vi "Append List to Report.vi"(0 "report in":refnum<class "NI_report.lvclass">, 1 "ordered item type (default)":T1(ring), 2 "unordered item type (default)":enum16{"(default)", "disc", "square", "circle"}(ring), 7 "list elements":string[](array[string]), 9 "list type (ordered)":enum16{"unordered", "ordered"}(ring)=enum."ordered", 11 "error in (no error)":errorcluster, 12 "ordered start (1)":i32=1, 13 "bookmark (Word)":string) -> (4 "report out":refnum<class "NI_report.lvclass">, 8 "start out (Word)":i32, 10 "end out (Word)":i32, 15 "error out":errorcluster)   [LabVIEW 2015, in "NI_report.lvclass"]
doc: "Adds a list of elements to the report."
uses:
  <vilib>/Utility/NIReport.llb/NI_report.lvclass
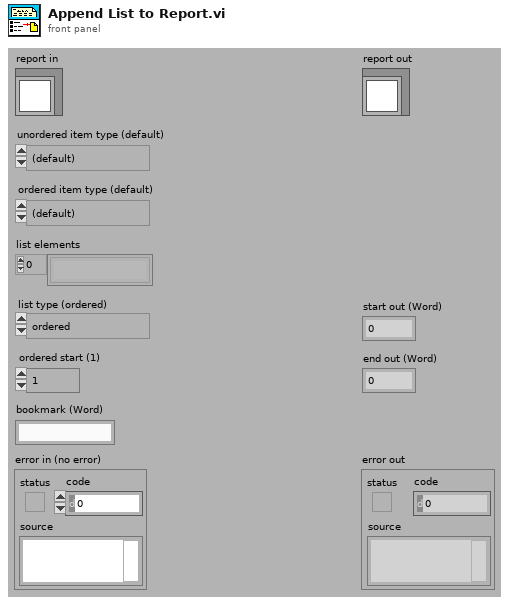
[diagram p1: front panel]
types:
  T1 = enum16{"(default)", "arabic numerals", "lower alpha", "upper alpha"}
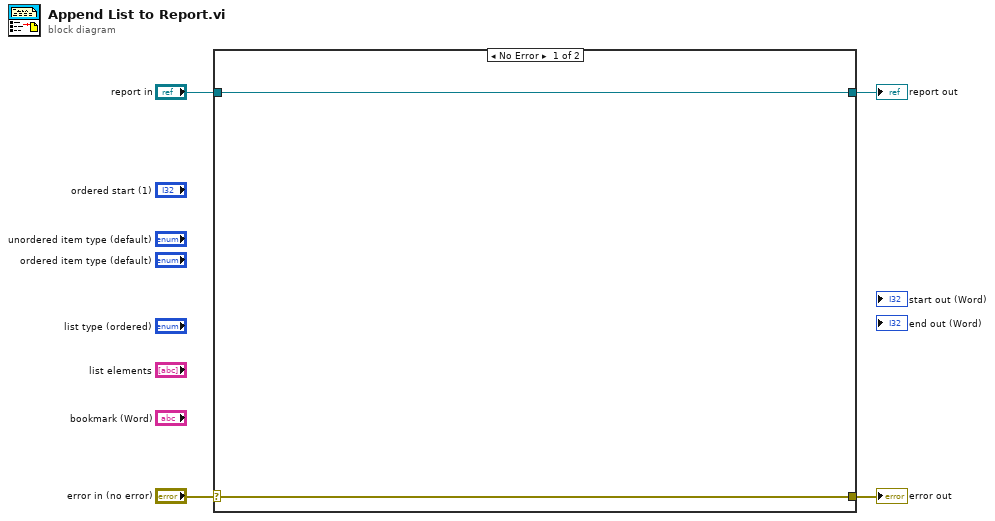
[diagram p0: block diagram]
diagram:
  n1 = case shown="No Error" "error in (no error)" {
    selector: "error in (no error)" -> [w5 w8]
    tunnel: [w5 w8] -> w3
    tunnel: [w6 w7] -> w1
    tunnel: "report in" -> [w6 w7]
    frame No Error {
    }
    frame Error {
    }
  }
  "error out" <- w3
  "report out" <- w1
